vi "WAPIAerSoftwareInitialize.vi"(0 "lpsParam":path, 9 "error in (no error)":errorcluster) -> (6 "error out":errorcluster)   [LabVIEW 2009]
uses:
  win50032.dll
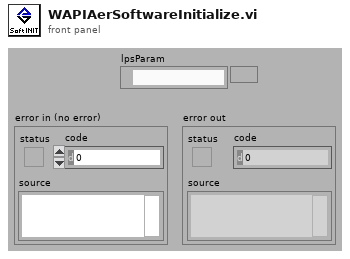
[diagram p1: front panel]
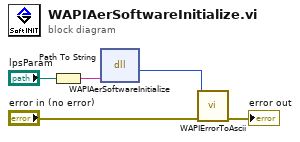
[diagram p0: block diagram]
diagram:
  n1 = Path To String(path="lpsParam") -> (string=w1:string)
  n2 = dll-call lib="Win50032.dll" fn="WAPIAerSoftwareInitialize"("lpsParam"=w1) -> ("return type"=w5:u32)  [unwired: 4 in, 2 out]
  n3 = call "WAPIErrorToAscii.vi"("error in (no error)"="error in (no error)", "error"=w5) -> ("error out"=→"error out":errorcluster)  [unwired: 8 in, 1 out]
